vi "PMUParse_90-5.vi"(8 "error in (no error)":errorcluster, 11 "DUT Data Row":u8[](array[numeric])=[1, 64, 162, 24, 128, 22, 0, 0, 0, 159, 0, 17, 92, 230, 0, 1, 0, 0, 0, 0, 0, 0, 0, 0, 0, 0, 0, 0, 0, 0, 0, 137, 130, 0, 64, 0, 0, 131, 96, 130, 0, 127, 128, 1, 1, 162, 130, 0, 120, 48, 130, 0, 116, 128, 11, 77, 83, 86, 73, 68, 32, 49, 45, 49, 45, 80, 130, 2, 0, 13, 131, 4, 0, 0, 0, 33, 132, 8, 71, 241, 43, 119, 55, 119, 119, 0, 133, 1, 1, 135, 130, 0, 76, 0, 64, 0, 0, 0, 0, 59, 52, 0, 0, 0, 0, 0, 0, 59, 52, 0, 0, 0, 0, 0, 0, 59, 52, 0, 0, 0, 0, 0, 0, 59, 52, 0, 0, 0, 0, 0, 0, 59, 52, 0, 0, 0, 0, 0, 0, 59, 52, 0, 0, 0, 0, 0, 0, 59, 52, 0, 0, 0, 0, 0, 0, 59, 52, 0, 0, 66, 112, 0, 0, 0, 0, 0, 0, 0, 0] format="%x") -> (0 "error out":errorcluster, 1 "PMUDataType":T1, 2 "MsgVersion":u8, 3 "PktData out":u8[](array[numeric]) format="%x", 5 "SyncOK":bool)   [LabVIEW 2014, in "SensorPlugins.lvlib" / "PmuBase.lvclass"]
uses:
  PmuBase.lvclass
  Typedef/PMUDataType.ctl
panel:
  out "time stamp size":u8
  out "Location of Time Stamp":u8
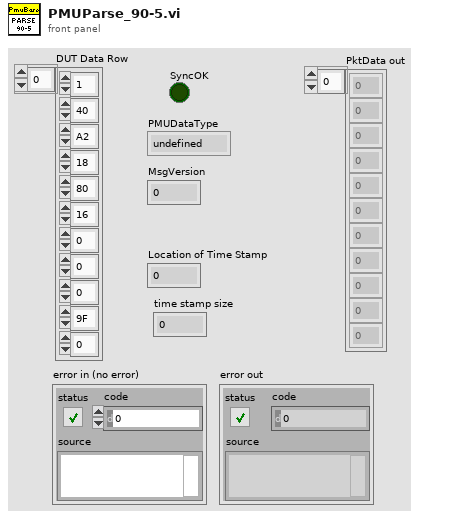
[diagram p1: front panel]
types:
  T1 = typedef "SensorPlugins.lvlib/PmuBase.lvclass/PMUDataType.ctl" = enum16{"undefined", "data", "header", "config 1", "config 2", "config 3", "command"}
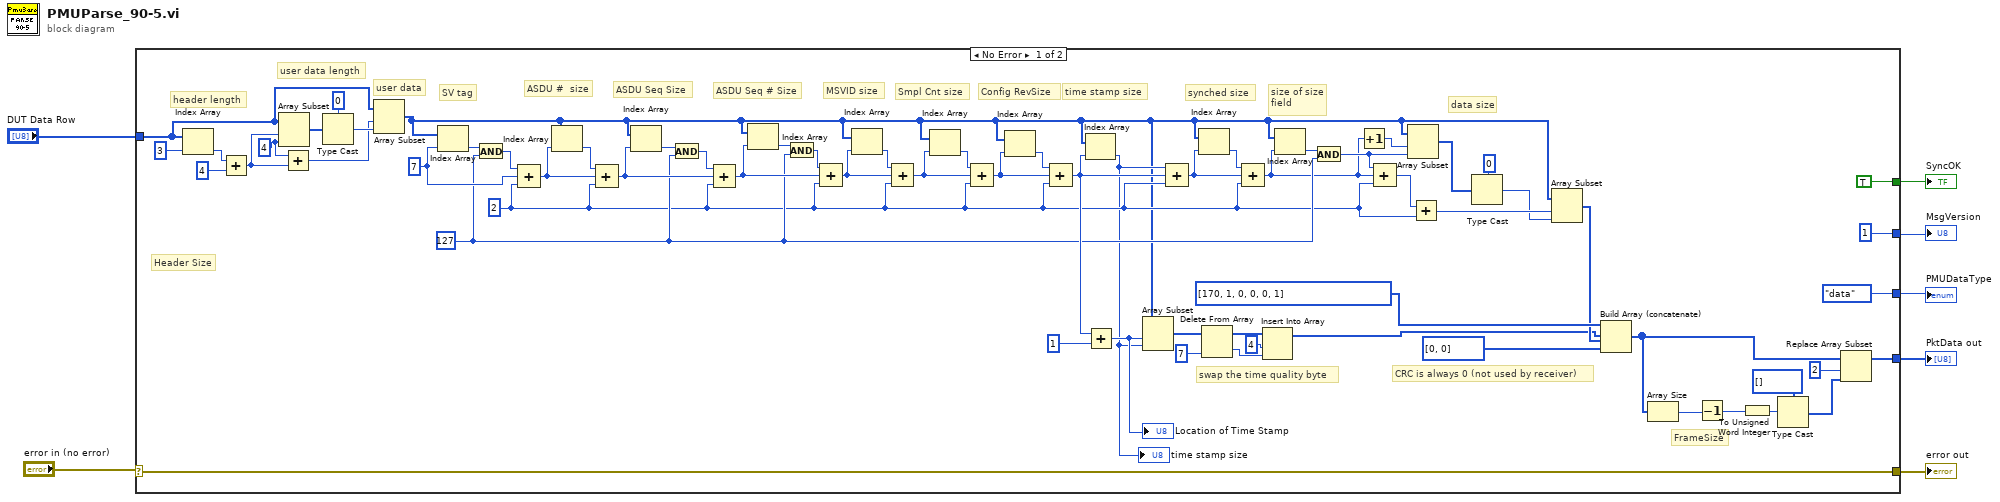
[diagram p0: block diagram]
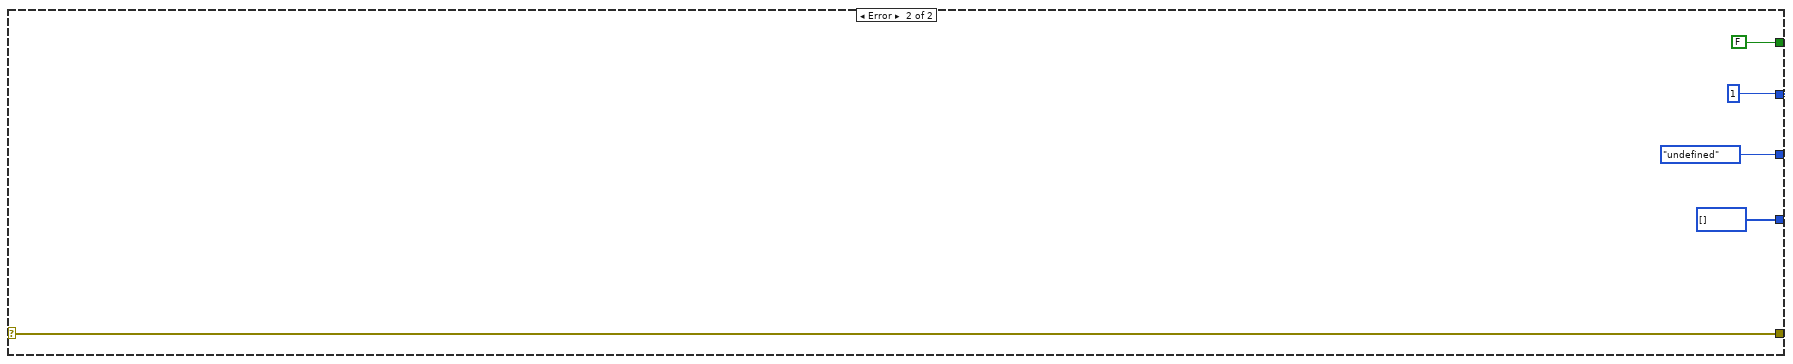
[diagram p2: hidden frame]
diagram:
  n1 = case shown="No Error" "error in (no error)" {
    selector: "error in (no error)" -> [w73 w78]
    tunnel: [w73 w78] -> w6
    tunnel: "DUT Data Row" -> [w67 _]
    tunnel: [w18 u8[] []] -> w4
    tunnel: [TRUE ("SyncOK") FALSE ("SyncOK")] -> w3
    tunnel: [u8 1 u8 1] -> w2
    tunnel: [PMUDataType."data" ("PMUDataType") PMUDataType."undefined" ("PMUDataType")] -> w1
    frame No Error {
      w38 = u8 2 ("value")
      w40 = u8 127
      w61 = u8 7 ("index")
      w64 = 4 ("length")
      # "swap the time quality byte"
      # "FrameSize"
      # "data size"
      # "CRC is always 0 (not used by receiver)"
      # "size of size\nfield"
      # "synched size"
      # "time stamp size"
      # "Config RevSize"
      # "Smpl Cnt size"
      # "MSVID size"
      # "ASDU Seq # Size"
      # "ASDU Seq Size"
      # "ASDU #  size"
      # "SV tag"
      # "user data"
      # "user data length"
      # "header length"
      # "Header Size"
      n2 = Index Array(array=w67, index=3) -> (element=w71:u8)
      n3 = Add(x=w71, y=u8 4) -> (x+y=w65:u8)
      n4 = Array Subset(array=w67, index=w65, length=w64) -> (w69:u8[])
      n5 = Add(x=w64, y=w65) -> (x+y=w63:i32)
      n6 = Type Cast(type=u32 0, x=w69) -> (*(type *) &x=w66:u32)
      n7 = Array Subset(array=w67, index=w63, length=w66) -> (w28:u8[])
      n8 = Index Array(array=w28, index=w61) -> (element=w62:u8)
      n9 = And(x=w62, y=w40) -> (x .and. y?=w60:u8)
      n10 = Compound Arithmetic op=ADD(w60, w61, w38) -> (w59:u8)
      n11 = Index Array(array=w28, index=w59) -> (element=w58:u8)
      n12 = Compound Arithmetic op=ADD(w58, w59, w38) -> (w55:u8)
      n13 = Index Array(array=w28, index=w55) -> (element=w57:u8)
      n14 = And(x=w57, y=w40) -> (x .and. y?=w56:u8)
      n15 = Compound Arithmetic op=ADD(w56, w55, w38) -> (w53:u8)
      n16 = Index Array(array=w28, index=w53) -> (element=w54:u8)
      n17 = And(x=w54, y=w40) -> (x .and. y?=w52:u8)
      n18 = Compound Arithmetic op=ADD(w52, w53, w38) -> (w50:u8)
      n19 = Index Array(array=w28, index=w50) -> (element=w51:u8)
      n20 = Compound Arithmetic op=ADD(w51, w50, w38) -> (w49:u8)
      n21 = Index Array(array=w28, index=w49) -> (element=w48:u8)
      n22 = Compound Arithmetic op=ADD(w48, w49, w38) -> (w47:u8)
      n23 = Index Array(array=w28, index=w47) -> (element=w46:u8)
      n24 = Compound Arithmetic op=ADD(w46, w47, w38) -> (w44:u8)
      n25 = Index Array(array=w28, index=w44) -> (element=w33:u8)
      "time stamp size" <- w33
      n26 = Add(x=w44, y=u8 1) -> (x+y=w34:u8)
      "Location of Time Stamp" <- w34
      n27 = Array Subset(array=w28, index=w34, length=w33) -> (w13:u8[])
      n28 = Compound Arithmetic op=ADD(w33, w44, w38) -> (w42:u8)
      n29 = Index Array(array=w28, index=w42) -> (element=w43:u8)
      n30 = Delete From Array(array=w13, index=7) -> (deleted portion=w10:u8, array with subset deleted=w11:u8[])  [unwired: 1 in]
      n31 = Compound Arithmetic op=ADD(w43, w42, w38) -> (w36:u8)
      n32 = Insert Into Array(array=w11, index=4, new element=w10) -> (w8:u8[])
      n33 = Index Array(array=w28, index=w36) -> (element=w41:u8)
      n34 = And(x=w41, y=w40) -> (x .and. y?=w37:u8)
      n35 = Increment(x=w36) -> (x+1=w35:u8)
      n36 = Compound Arithmetic op=ADD(w37, w36, w38) -> (w39:u8)
      n37 = Array Subset(array=w28, index=w35, length=w37) -> (w32:u8[])
      n38 = Add(x=w39, y=w38) -> (x+y=w30:u8)
      n39 = Type Cast(type=u32 0, x=w32) -> (*(type *) &x=w29:u32)
      n40 = Array Subset(array=w28, index=w30, length=w29) -> (w26:u8[])
      n41 = Build Array (concatenate)(u8[] [170, 1, 0, 0, 0, 1], w8, w26, u8[] [0, 0]) -> (w20:u8[])
      n42 = Array Size(array=w20) -> (size(s)=w25:i32)
      n43 = Decrement(x=w25) -> (x-1=w14:i32)
      n44 = To Unsigned Word Integer(number=w14) -> (unsigned 16bit integer=w23:u16)
      n45 = Type Cast(type=u8[] [], x=w23) -> (*(type *) &x=w21:u8[])
      n46 = Replace Array Subset(array=w20, new element=w21, index=2) -> (w18:u8[])
    }
    frame Error {
    }
  }
  "error out" <- w6
  "SyncOK" <- w3
  "MsgVersion" <- w2
  "PMUDataType" <- w1
  "PktData out" <- w4
